vi "Error Process.vi"(8 "error in (no error)":errorcluster, 11 "View Model":T1) -> (0 "error out":errorcluster)   [LabVIEW 2017]
doc: "Separate process for Error Handler of three predefined Error's levels.\n[Covers: EH1]"
uses:
  Model/Controls/View Model.ctl
  Model/Controls/Shared Model.ctl
  Model/Controls/Views Action.ctl
  Controls/Error Model.ctl
  Controls/Error Message.ctl
  Controls/Error Type.ctl
  Configuration/Controls/Config Model.ctl
  Configuration/Controls/Config DB Message.ctl
  Configuration/Controls/Config DB Command.ctl
  Configuration/Controls/Config DB Overhead.ctl
  Configuration/Controls/Config DB Record.ctl
  Controller/Controls/Controller Model.ctl
  Views/Vehicle Position Simulation View/Controls/Vehicle - Position.ctl
  Controller/Controls/Controller Overhead.ctl
  Controller/Controls/Controller Wash Step.ctl
  Controller/Controls/Controller State.ctl
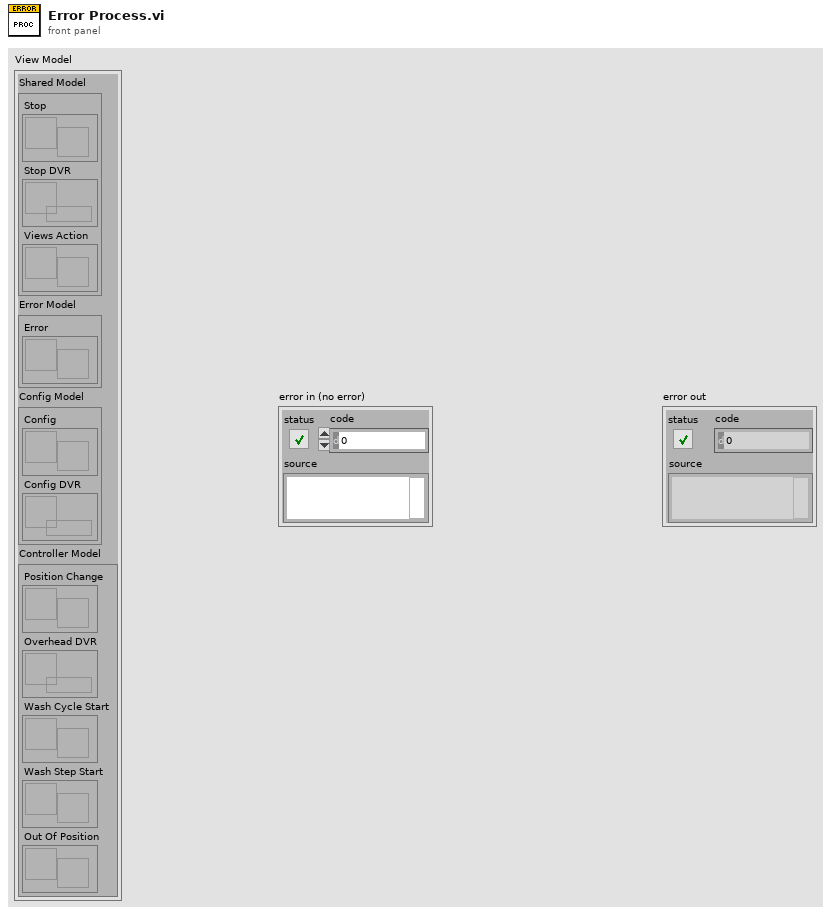
[diagram p1: front panel]
types:
  T1 = typedef "View Model.ctl" = cluster{"Shared Model":T2, "Error Model":T3, "Config Model":T4, "Controller Model":T5}
  T2 = typedef "Shared Model.ctl" = cluster{"Stop":refnum<user-event>, "Stop DVR":refnum<data-value>, "Views Action":refnum<user-event>}
  T3 = typedef "Error Model.ctl" = cluster{"Error":refnum<user-event>}
  T4 = typedef "Config Model.ctl" = cluster{"Config":refnum<user-event>, "Config DVR":refnum<data-value>}
  T5 = typedef "Controller Model.ctl" = cluster{"Position Change":refnum<user-event>, "Overhead DVR":refnum<data-value>, "Wash Cycle Start":refnum<user-event>, "Wash Step Start":refnum<user-event>, "Out Of Position":refnum<user-event>}
  T6 = typedef "Error Type.ctl" = enum16{"Minor Error", "Wash Cycle Error", "System Error", "Unknown"}
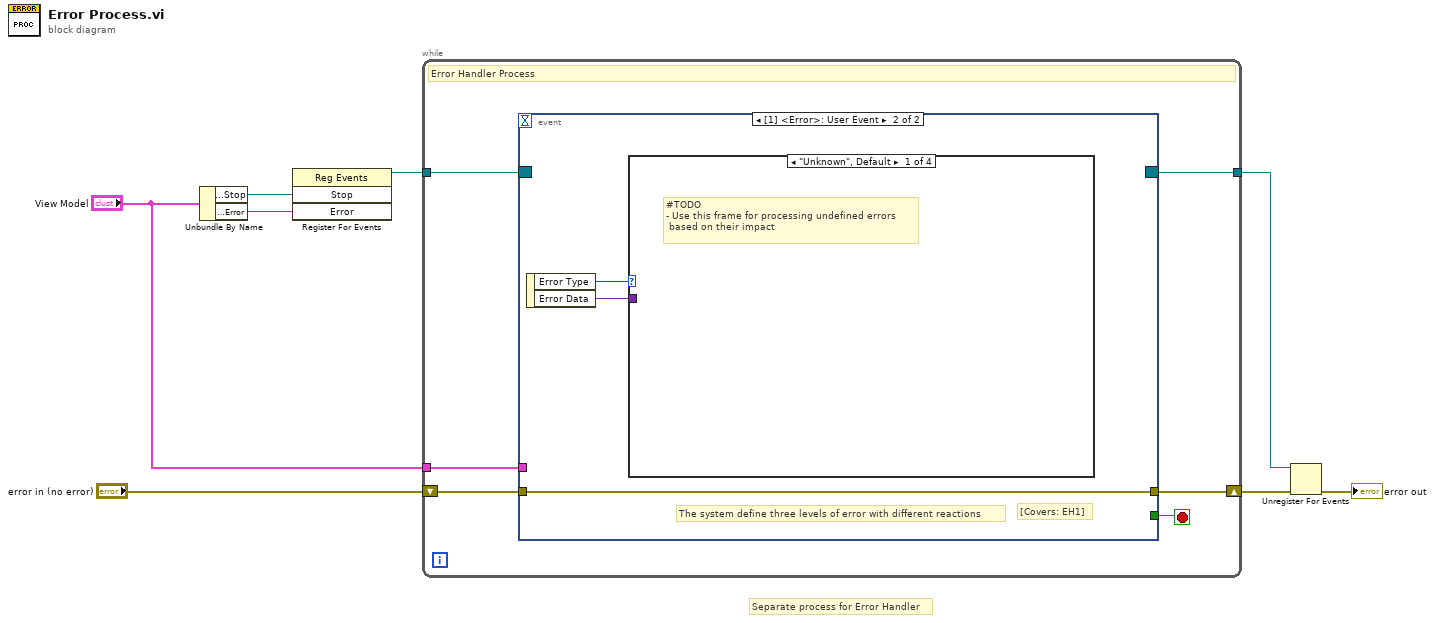
[diagram p0: block diagram]
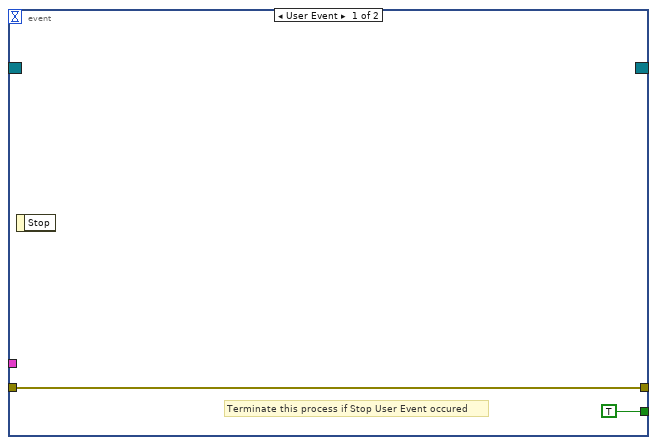
[diagram p2: hidden frame]
diagram:
  # "Separate process for Error Handler"
  n1 = Unbundle By Name("View Model") -> ("Shared Model.Stop"=w8:refnum<user-event>, "Error Model.Error"=w1:refnum<user-event>)
  n2 = register-events(w8, w1) -> (reference out=w7:refnum<event-registration>)  [unwired: 2 in, 1 out]
  n3 = while {
    tunnel: w7 -> [w14]
    shift-right: [w12] -> w5
    shift-left: "error in (no error)" -> [w13]
    tunnel: [w11] -> w3
    tunnel: "View Model" -> [w10]
    stop <- w9 stop-if-true
    # "Error Handler Process"
    n4 = event shown="[1] <Error>: User Event" {
      selector: w14 -> [_ _]
      dyn-events: [_ _] -> w11
      timeout: _ -> [_ _]
      tunnel: w13 -> [w16 w19]
      tunnel: [w16 w19] -> w12
      tunnel: w10 -> [_ _]
      tunnel: [TRUE _] -> w9
      event User Event {
        # "Terminate this process if Stop User Event occured"
        n5 = event-data() -> ()  [unwired: 1 in, 1 out]
      }
      event User Event {
        # "The system define three levels of error with different reactions"
        # "[Covers: EH1]"
        n6 = event-data() -> ("Error Type"=w18:T6, "Error Data"=w17:variant)  [unwired: 1 in]
        n7 = case shown="\"Unknown\", Default" w18 {
          tunnel: w17 -> [_ _ _ _]
          frame "Unknown", Default {
            # "#TODO\n- Use this frame for processing undefined errors\n based on their impact"
          }
          frame "Minor Error" {
            # "[Covers: EH1B]"
            # "#TODO\nMake this error type invicible for user.\nClear Error and continue any operation without interruption."
          }
          frame "Wash Cycle Error" {
            # "[Covers: EH1B2]"
            # "[Covers: EH1B1]"
            # "[Covers: EH1B]"
            # "#TODO\n- Set next state DVR = Wash Abort/Terminate.\n- Display Error Dialog for user to move car to the Exit position.\n- Reinit CarWash controller for new cycle."
          }
          frame "System Error" {
            # "[Covers: EH1C3]"
            # "[Covers: EH1C2]"
            # "[Covers: EH1C1]"
            # "[Covers: EH1C]"
            # "#TODO\n- Set next state DVR = Wash Abort/Terminate.\n- Display Error Dialog for user to move car to the Exit position.\n- Generate Stop User Event for all UI and HW. Terminate App."
          }
        }
      }
    }
  }
  n8 = Unregister For Events(event registration refnum=w3, error in=w5) -> (error out=→"error out":errorcluster)
